vi "Process (SRAM 64-Bit).vi"(0 "write data":T5, 1 "reset":bool, 2 "resources":T1={"io resources"={"address"="SRAM\\Address", "read"="SRAM\\Command", "input valid"="SRAM\\Push_Fifo", "write data"="SRAM\\Write_Data", "read data"="SRAM\\Read_Data", "read data valid"="SRAM\\Read_Data_Valid", "ready for input"="SRAM\\Fifo_Full"}}, 5 "read request":T4, 12 "ready for retrieve data (T)":bool=TRUE) -> (3 "in reset":bool, 4 "retrieve data":T3, 13 "ready for read request":bool, 14 "ready for write":bool)   [LabVIEW 2012, in "FIFO.lvlib" / "niRFRIO Memory 1.0.0 FPGA.lvlib"]
uses:
  <userlib>/FPGA Library/Code Development/DRAM/RF-RIO/Memory/1.0.0/FPGA/niRFRIO Memory 1.0.0 FPGA.lvlib
  <userlib>/FPGA Library/Code Development/DRAM/RF-RIO/Memory/1.0.0/FPGA/Public/Write Data (64-Bit No Byte Enables).ctl
  <userlib>/FPGA Library/Code Development/DRAM/RF-RIO/Memory/1.0.0/FPGA/Public/Read Request.ctl
  <userlib>/FPGA Library/Code Development/DRAM/RF-RIO/Memory/1.0.0/FPGA/Public/Retrieve Data (64-Bit).ctl
  <userlib>/FPGA Library/Code Development/DRAM/RF-RIO/SRAM/1.0.0/FPGA/Public/Resources.ctl
  <userlib>/FPGA Library/Code Development/DRAM/RF-RIO/SRAM/1.0.0/FPGA/Public/IO Resources.ctl
  <userlib>/FPGA Library/Code Development/DRAM/RF-RIO/SRAM/1.0.0/FPGA/niRFRIO SRAM 1.0.0 FPGA.lvlib
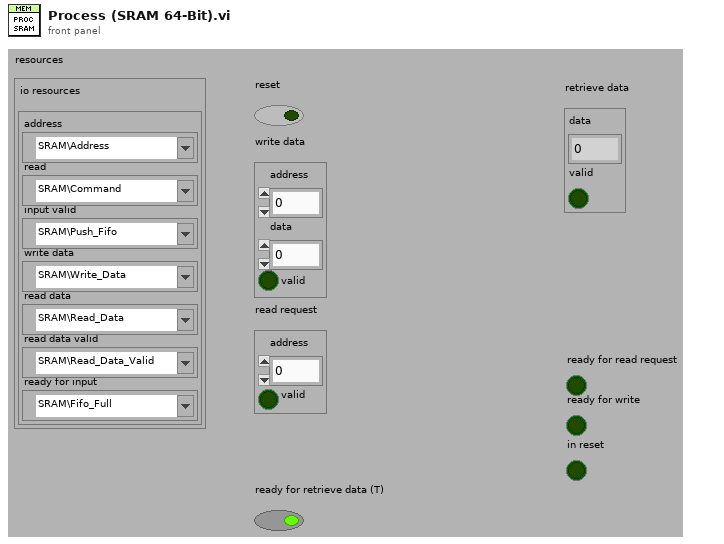
[diagram p1: front panel]
types:
  T1 = typedef "niRFRIO SRAM 1.0.0 FPGA.lvlib/Resources.ctl" = cluster{"io resources":T2}
  T2 = typedef "niRFRIO SRAM 1.0.0 FPGA.lvlib/IO Resources.ctl" = cluster{"address":refnum<k21>, "read":refnum<k21>, "input valid":refnum<k21>, "write data":refnum<k21>, "read data":refnum<k21>, "read data valid":refnum<k21>, "ready for input":refnum<k21>}
  T3 = typedef "FIFO.lvlib/niRFRIO Memory 1.0.0 FPGA.lvlib/Retrieve Data (64-Bit).ctl" = cluster{"data":u64, "valid":bool}
  T4 = typedef "FIFO.lvlib/niRFRIO Memory 1.0.0 FPGA.lvlib/Read Request.ctl" = cluster{"address":u32, "valid":bool}
  T5 = typedef "FIFO.lvlib/niRFRIO Memory 1.0.0 FPGA.lvlib/Write Data (64-Bit No Byte Enables).ctl" = cluster{"address":u32, "data":u64, "valid":bool}
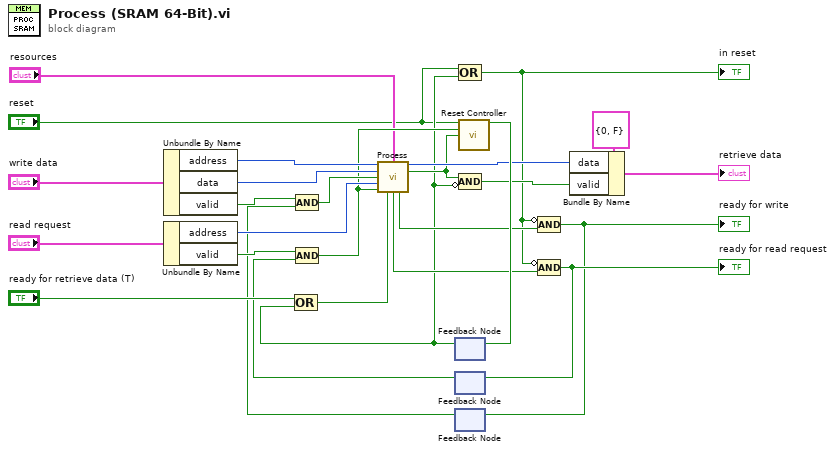
[diagram p0: block diagram]
diagram:
  n1 = Unbundle By Name("write data") -> ("address"=w17:u32, "data"=w16:u64, "valid"=w21:bool)
  n2 = Unbundle By Name("read request") -> ("address"=w10:u32, "valid"=w9:bool)
  n3 = feedback #1() -> (w3:bool)  [unwired: 1 in]
  n4 = Compound Arithmetic op=OR("ready for retrieve data (T)", w3) -> (w12:bool)
  n5 = feedback #2() -> (w7:bool)  [unwired: 1 in]
  n6 = Compound Arithmetic op=AND(w9, w7) -> (w8:bool)
  n7 = feedback #3() -> (w6:bool)  [unwired: 1 in]
  n8 = Compound Arithmetic op=AND(w21, w6) -> (w15:bool)
  n9 = call <userlib>:"Process.vi"("write address"=w17, "resources"="resources", "write data"=w16, "write data valid"=w15, "read address"=w10, "read address valid"=w8, "ready for retrieve data (T)"=w12) -> ("retrieve data"=w13:u64, "retrieve data valid"=w4:bool, "ready for read request"=w11:bool, "ready for write"=w14:bool)  [unwired: 5 in]
  n10 = Compound Arithmetic op=OR("reset", w3) -> (w1:bool)
  "in reset" <- w1
  n11 = call <userlib>:"Reset Controller.vi"("reset"="reset", "issued read request"=w8, "retrieved data"=w4) -> ("flushing memory pipe"=w20:bool)  [unwired: 12 in]
  n12 = feedback-in #1(w20) -> ()
  n13 = Compound Arithmetic op=AND(w4, invert w3) -> (w18:bool)
  n14 = Compound Arithmetic op=AND(invert w1, w14) -> (w22:bool)
  "ready for write" <- w22
  n15 = feedback-in #3(w22) -> ()
  n16 = Compound Arithmetic op=AND(invert w1, w11) -> (w23:bool)
  "ready for read request" <- w23
  n17 = feedback-in #2(w23) -> ()
  n18 = Bundle By Name(cluster=T3 {"data"=0, "valid"=FALSE} ("retrieve data"), "data"=w13, "valid"=w18) -> (→"retrieve data":T3)
